vi "Бегущие лампочки.vi"() -> ()   [LabVIEW 2017]
panel:
  out "4":bool
  out "3":bool
  out "2":bool
  out "1":bool
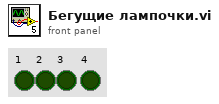
[diagram p1: front panel]
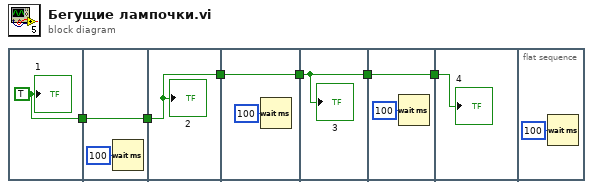
[diagram p0: block diagram]
diagram:
  n1 = flat-sequence {
    tunnel: [w7] -> w6
    tunnel: w6 -> [w8]
    tunnel: [w8] -> w5
    tunnel: w5 -> [w10]
    tunnel: [w10] -> w4
    tunnel: w4 -> [w11]
    tunnel: [w11] -> w3
    tunnel: w3 -> [w13]
    tunnel: [w13] -> w2
    tunnel: w2 -> [w14]
    tunnel: [w14] -> w1
    tunnel: w1 -> [w16]
    frame #0 {
      w7 = TRUE ("1")
      "1" <- w7
    }
    frame #1 {
      n2 = Wait (ms)(milliseconds to wait=u32 100) -> ()  [unwired: 1 out]
    }
    frame #2 {
      "2" <- w10
    }
    frame #3 {
      n3 = Wait (ms)(milliseconds to wait=u32 100) -> ()  [unwired: 1 out]
    }
    frame #4 {
      "3" <- w13
    }
    frame #5 {
      n4 = Wait (ms)(milliseconds to wait=u32 100) -> ()  [unwired: 1 out]
    }
    frame #6 {
      "4" <- w16
    }
    frame #7 {
      n5 = Wait (ms)(milliseconds to wait=u32 100) -> ()  [unwired: 1 out]
    }
  }
